vi "CRYFlatten Stimulus Element.vi"(8 "Stimulus Type":T1 items=["Frequency Stepped Sweep", "Frequency Log Sweep", "Log Amplitude Sweep", "WAV", "DC Connect", "Two Tone", "Noise", "Multitone"], 11 "Flattened Stimulus Element":string) -> (3 "Flatten Stimulus Setup String":string)   [LabVIEW 2013]
uses:
  Typedef Control/CRYStimulus Type.ctl
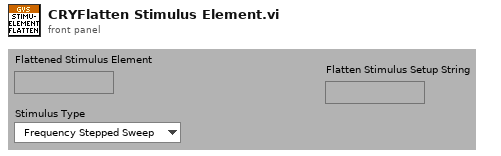
[diagram p1: front panel]
types:
  T1 = typedef "CRYStimulus Type.ctl" = u16
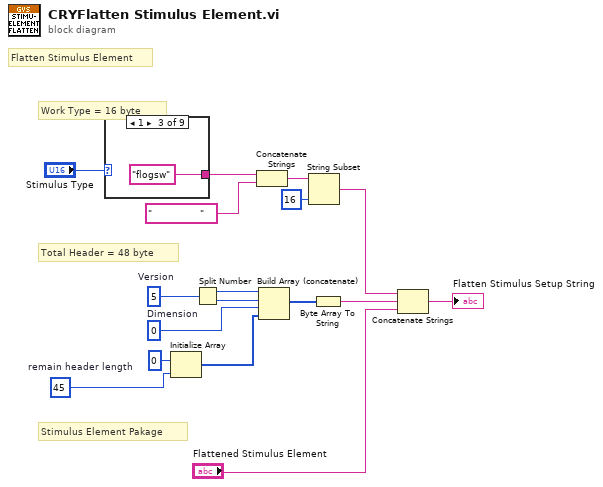
[diagram p0: block diagram]
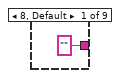
[diagram p2: hidden frame]
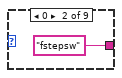
[diagram p3: hidden frame]
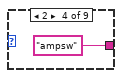
[diagram p4: hidden frame]
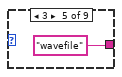
[diagram p5: hidden frame]
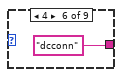
[diagram p6: hidden frame]
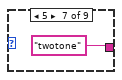
[diagram p7: hidden frame]
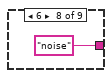
[diagram p8: hidden frame]
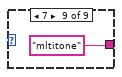
[diagram p9: hidden frame]
diagram:
  w12 = u16 5  # Version
  w9 = u8 0  # Dimension
  w13 = 45  # remain header length
  # "Flatten Stimulus Element"
  # "Stimulus Element Pakage"
  # "Work Type = 16 byte"
  # "Total Header = 48 byte"
  n1 = case shown="1" "Stimulus Type" {
    tunnel: ["" ("string") "fstepsw" ("string") "flogsw" ("string") "ampsw" ("string") "wavefile" ("string") "dcconn" ("string") "twotone" ("string") "noise" ("string") "mltitone" ("string")] -> w2
    frame 8, Default {
    }
    frame 0 {
    }
    frame 1 {
    }
    frame 2 {
    }
    frame 3 {
    }
    frame 4 {
    }
    frame 5 {
    }
    frame 6 {
    }
    frame 7 {
    }
  }
  n2 = Initialize Array(u8 0 ("element"), w13) -> (w7:u8[])
  n3 = Split Number(x=w12) -> (hi(x)=w11:u8, lo(x)=w10:u8)
  n4 = Concatenate Strings(w2, "                " ("string")) -> (w16:string)
  n5 = Build Array (concatenate)(w11, w10, w9, w7) -> (w8:u8[])
  n6 = String Subset(string=w16, length (rest)=16 ("length (rest)")) -> (substring=w5:string)  [unwired: 1 out]
  n7 = Byte Array To String(unsigned byte array=w8) -> (string=w6:string)
  n8 = Concatenate Strings(w5, w6, "Flattened Stimulus Element") -> (→"Flatten Stimulus Setup String":string)
